vi "Access Privilege_LV2G_Privilege.vi"(6 "User Name":string, 7 "Verified":bool, 8 "error in (no error)":errorcluster, 9 "Password in":string, 10 "Privillage":string, 11 "Actions":enum16{"Read", "Write", "Initialize"}(ring)) -> (0 "error out":errorcluster, 1 "Password out":string, 2 "Verified out":bool, 3 "Privillage Out":string, 4 "User Name":string)   [LabVIEW 2023, in "GUI.lvlib"]
uses:
  GUI.lvlib
panel:
  # "Input to this VI"
  # "Output from this VI"
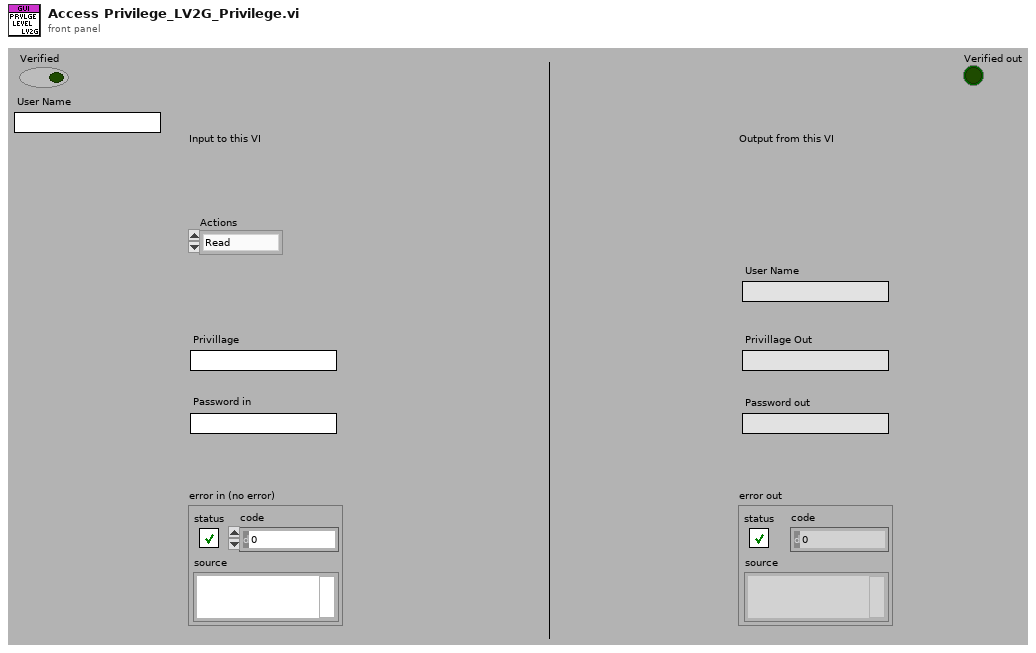
[diagram p1: front panel]
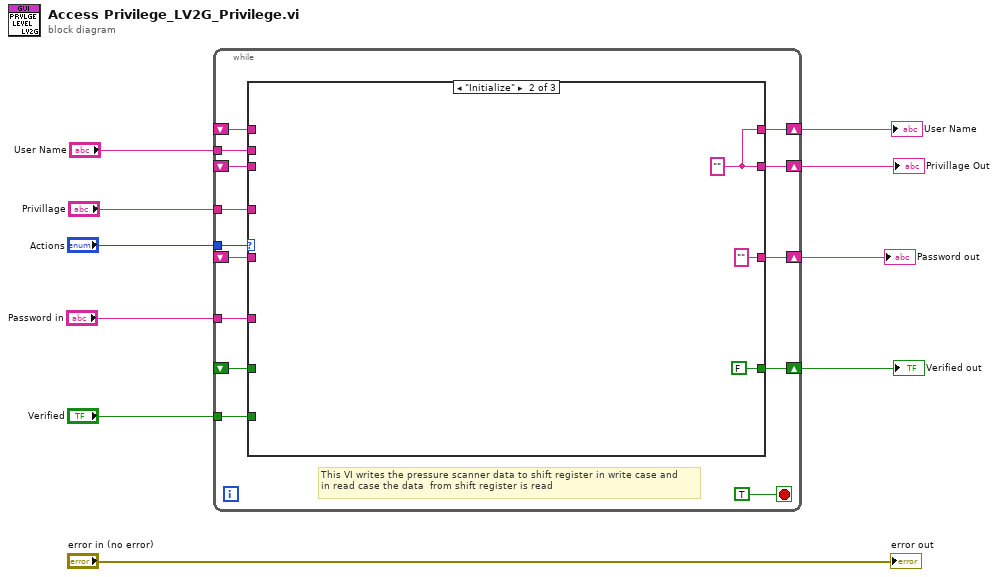
[diagram p0: block diagram]
diagram:
  n1 = while {
    tunnel: "Actions" -> [w23]
    shift-right: [w22] -> w8
    shift-left: _ -> [w20]
    tunnel: "Privillage" -> [w21]
    tunnel: "Password in" -> [w18]
    shift-right: [w19] -> w6
    shift-left: _ -> [w17]
    shift-right: [w16] -> w3
    shift-left: _ -> [w14]
    tunnel: "Verified" -> [w15]
    shift-right: [w12] -> w2
    shift-left: _ -> [w13]
    tunnel: "User Name" -> [w11]
    stop <- TRUE stop-if-true
    # "This VI writes the pressure scanner data to shift register in write case and\nin read case the data  from shift register is read"
    n2 = case shown="\"Initialize\"" w23 {
      tunnel: [w28 w29 w35] -> w22
      tunnel: w21 -> [_ _ w35]
      tunnel: w20 -> [w28 _ _]
      tunnel: [w27 "" ("UserName in") w34] -> w19
      tunnel: w18 -> [_ _ w34]
      tunnel: w17 -> [w27 _ _]
      tunnel: [w26 FALSE w33] -> w16
      tunnel: w15 -> [_ _ w33]
      tunnel: w14 -> [w26 _ _]
      tunnel: [w25 w29 w32] -> w12
      tunnel: w13 -> [w25 _ _]
      tunnel: w11 -> [_ _ w32]
      frame "Read", Default {
      }
      frame "Initialize" {
        w29 = "" ("String")
      }
      frame "Write" {
      }
    }
  }
  "Privillage Out" <- w8
  "Password out" <- w6
  "Verified out" <- w3
  "User Name" <- w2
  "error out" <- "error in (no error)"
